vi "Reader API.vi"(0 "COM":refnum<visa-resource-name>, 1 "Baudrate":u32=19200, 2 "Timeout (ms)":u32=500, 5 "Function":string(combo), 7 "Address":string="X", 11 "error in (no error)":errorcluster, 12 "COM Port Type":T1(ring)=enum."SendWaitRead", 13 "REC":string) -> (4 "ReceiveString":string, 6 "Return":string, 8 "pass?":bool, 15 "error out":errorcluster)   [LabVIEW 2020]
uses:
  UART/UART.lvlib
panel:
  out "ID output":string
  in  "Data":string
  # "NOTICE -- YOU MUST LEAVE THIS NOTICE IN PLACE.\n\nCopyright (c) 2017, Fred Guo Guohuijun0422@Gmail.com All rights reserved."
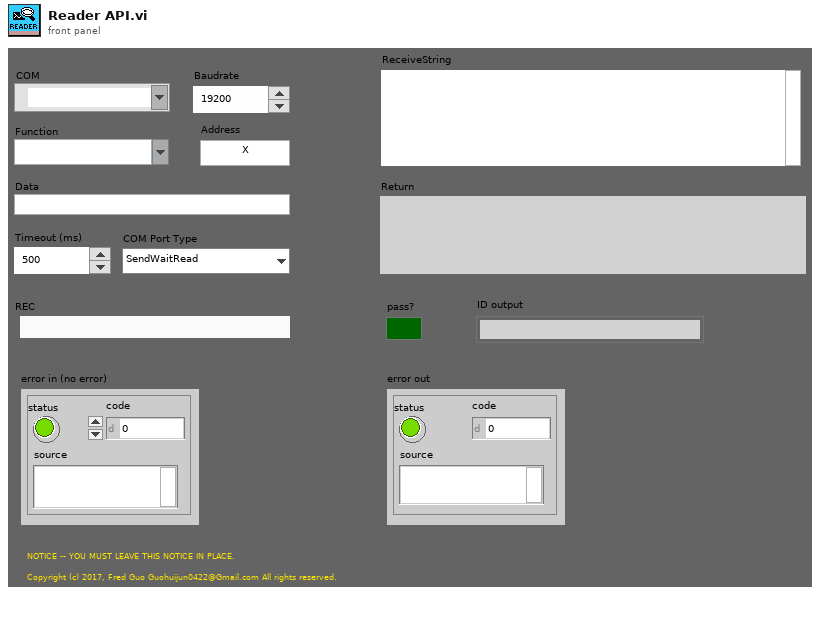
[diagram p1: front panel]
types:
  T1 = enum16{"Open", "Close", "ClearBuffer", "Send", "Read", "SendWaitRead", "SendCompare", "ReadCompare"}
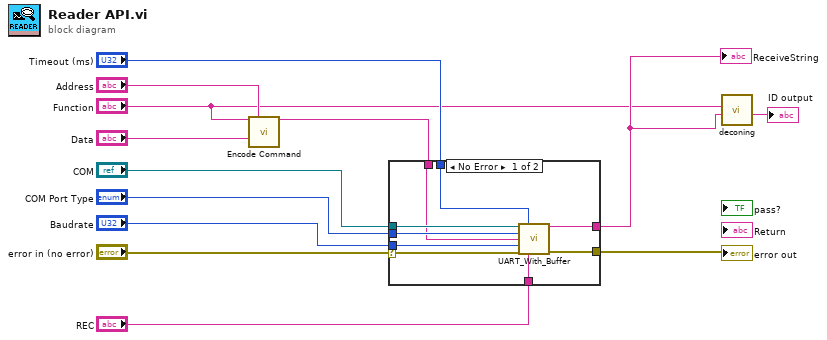
[diagram p0: block diagram]
diagram:
  n1 = call "Encode Command.vi"("Function"="Function", "Address"="Address", "Data"="Data") -> ("Command out"=w13:string)  [unwired: 12 in]
  n2 = case shown="No Error" "error in (no error)" {
    selector: "error in (no error)" -> [w19 w23]
    tunnel: w13 -> [w15 _]
    tunnel: "COM" -> [w22 _]
    tunnel: "Timeout (ms)" -> [w14 _]
    tunnel: "COM Port Type" -> [w21 _]
    tunnel: "Baudrate" -> [w20 _]
    tunnel: "REC" -> [w18 _]
    tunnel: [w17 _] -> w3
    tunnel: [w16 w23] -> w4
    frame No Error {
      n3 = call "UART_With_Buffer.vi"("COM"=w22, "Timeout (ms)"=w14, "Function"=w21, "Send"=w15, "Baudrate"=w20, "error in (no error)"=w19, "Read regular"=w18) -> ("ReceiveString"=w17:string, "error out"=w16:errorcluster)  [unwired: 7 in]
    }
    frame Error {
    }
  }
  "ReceiveString" <- w3
  "error out" <- w4
  n4 = call "deconing.vi"("Hex input"=w3, "Function"="Function") -> ("ID output"=→"ID output":string)  [unwired: 9 in]
